vi "16-CalculateVersionSum.vi"(10 "Packet in":T1) -> (1 "Version Sum":u32, 2 "Packet out":T1)   [LabVIEW 2019, in "16.lvlib"]
uses:
  16.lvlib
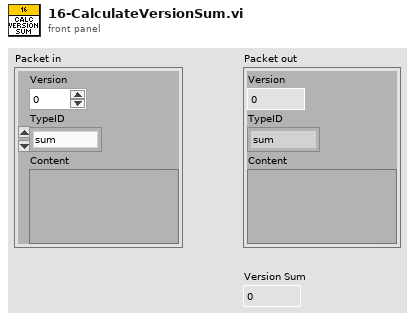
[diagram p1: front panel]
types:
  T1 = cluster{"Version":u32, "TypeID":enum16{"sum", "product", "minimum", "maximum", "literal", "greater than", "less than", "equal to"}, "Content":variant}
  T2 = enum16{"sum", "product", "minimum", "maximum", "literal", "greater than", "less than", "equal to"}
  T3 = cluster{"Version":u32, "TypeID":enum16{"sum", "product", "minimum", "maximum", "literal", "greater than", "less than", "equal to"}, "Content":variant}[]
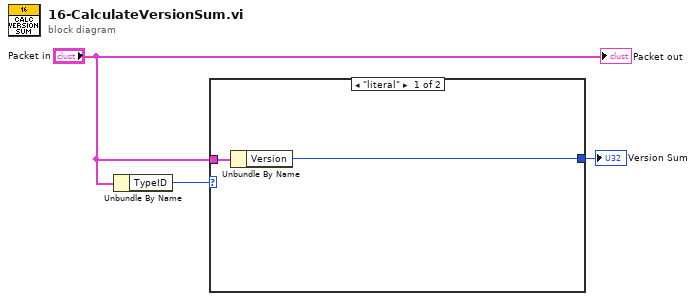
[diagram p0: block diagram]
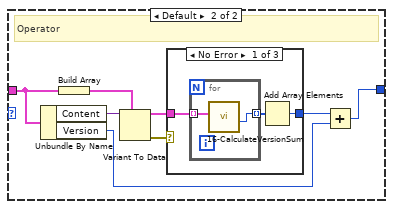
[diagram p2: hidden frame]
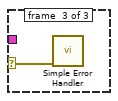
[diagram p4: hidden frame]
diagram:
  n1 = Unbundle By Name("Packet in") -> ("TypeID"=w1:T2)
  n2 = case shown="\"literal\"" w1 {
    tunnel: [w4 w9] -> w3
    tunnel: "Packet in" -> [w5 w12]
    frame "literal" {
      n3 = Unbundle By Name(w5) -> ("Version"=w4:u32)
    }
    frame Default {
      # "Operator"
      n4 = Unbundle By Name(w12) -> ("Content"=w13:variant, "Version"=w8:u32)
      n5 = Build Array(w12) -> (w11:T3)
      n6 = Variant To Data(type=w11, Variant=w13) -> (data=w10:T3, error out=w6:errorcluster)  [unwired: 1 in]
      n7 = case shown="No Error" w6 {
        selector: w6 -> [_ _ w19]
        tunnel: w10 -> [w16 _ _]
        tunnel: [w14 _ _] -> w7
        frame #0 {
          n8 = for {
            tunnel: w16 -> [w18] mode=indexing
            tunnel: [w17] -> w15 mode=indexing
            n9 = call "16-CalculateVersionSum.vi"("Packet in"=w18) -> ("Version Sum"=w17:u32)  [unwired: 9 in, 1 out]
          }
          n10 = Add Array Elements(numeric array=w15) -> (sum=w14:u32)
        }
        frame #1 {
          # "NULL Packet"
        }
        frame #2 {
          n11 = call <vilib>:"Simple Error Handler.vi"("error in (no error)"=w19) -> ()  [unwired: 4 in, 5 out]
        }
      }
      n12 = Add(x=w7, y=w8) -> (x+y=w9:u32)
    }
  }
  "Version Sum" <- w3
  "Packet out" <- "Packet in"
